vi "create icon from picdata.vi"(1 "image data":T1, 2 "Pict Refnum":refnum<vi>) -> (0 "new picture":picture)   [LabVIEW 2014, in "POLARIS IMAQ Display.xctl"]
uses:
  POLARIS IMAQ Display.xctl
  <vilib>/picture/picture.llb/imagedata.ctl
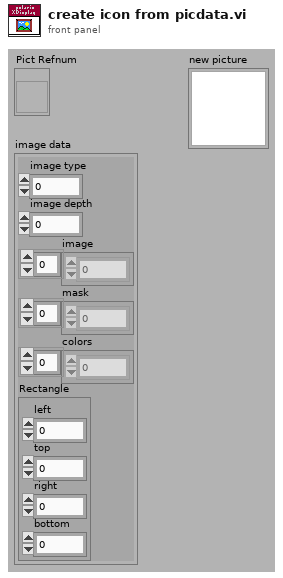
[diagram p1: front panel]
types:
  T1 = typedef "imagedata.ctl" = cluster{"image type":i32, "image depth":i32, "image":u8[], "mask":u8[], "colors":u32[], "Rectangle":cluster{"left":i16, "top":i16, "right":i16, "bottom":i16}}
  T2 = typedef "LVBoundsTypeDef.ctl" = cluster{"Width":u32, "Height":u32}
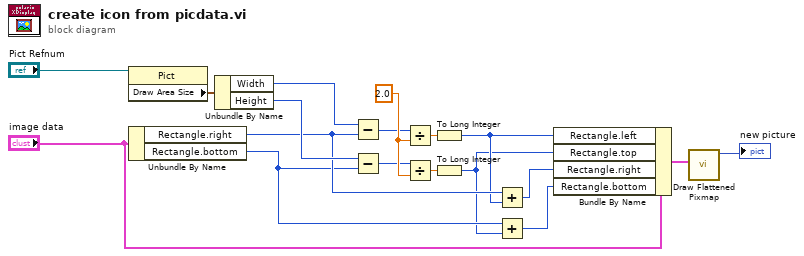
[diagram p0: block diagram]
diagram:
  w11 = 2.0 ("y")
  n1 = property on="Property Node" class="Pict"(reference="Pict Refnum") -> ("Draw Area Size"=w6:T2)  [unwired: 1 in, 2 out]
  n2 = Unbundle By Name("image data") -> ("Rectangle.right"=w4:i16, "Rectangle.bottom"=w3:i16)
  n3 = Unbundle By Name(w6) -> ("Width"=w7:u32, "Height"=w8:u32)
  n4 = Subtract(x=w7, y=w4) -> (x-y=w9:u32)
  n5 = Subtract(x=w8, y=w3) -> (x-y=w10:u32)
  n6 = Divide(x=w9, y=w11) -> (x/y=w12:dbl)
  n7 = Divide(x=w10, y=w11) -> (x/y=w14:dbl)
  n8 = To Long Integer(number=w12) -> (32bit integer=w2:i32)
  n9 = To Long Integer(number=w14) -> (32bit integer=w1:i32)
  n10 = Add(x=w4, y=w2) -> (x+y=w13:i32)
  n11 = Add(x=w3, y=w1) -> (x+y=w15:i32)
  n12 = Bundle By Name(cluster="image data", "Rectangle.left"=w2, "Rectangle.top"=w1, "Rectangle.right"=w13, "Rectangle.bottom"=w15) -> (w17:T1)
  n13 = call <vilib>:"Draw Flattened Pixmap.vi"("image data"=w17) -> ("new picture"=→"new picture":picture)  [unwired: 8 in]
